vi "Grow bounding rectangle N pixels.vi"(4 "Bounding Rect":T1={"Left"=20.0, "Top"=30.0, "Right"=200.0, "Bottom"=300.0}, 5 "# pixels":dbl=10.0) -> (1 "Bounding Rect expanded":T1={"Left"=10.0, "Top"=20.0, "Right"=210.0, "Bottom"=310.0})   [LabVIEW 2013]
doc: "Grows outwardeach side of bounding rectangle by N pixels."
uses:
  Project Vis/Image Analysis/Analysis type defs/Bounding rectangle cluster.ctl
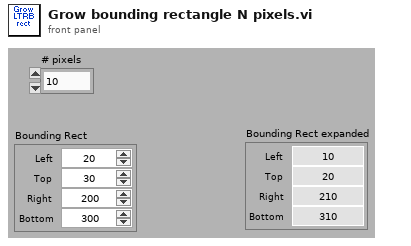
[diagram p1: front panel]
types:
  T1 = typedef "Bounding rectangle cluster.ctl" = cluster{"Left":dbl, "Top":dbl, "Right":dbl, "Bottom":dbl}
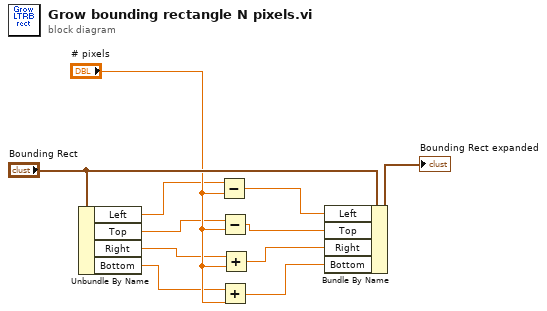
[diagram p0: block diagram]
diagram:
  n1 = Unbundle By Name("Bounding Rect") -> ("Left"=w8:dbl, "Top"=w7:dbl, "Right"=w6:dbl, "Bottom"=w5:dbl)
  n2 = Subtract(x=w8, y="# pixels") -> (x-y=w4:dbl)
  n3 = Subtract(x=w7, y="# pixels") -> (x-y=w3:dbl)
  n4 = Add(x=w5, y="# pixels") -> (x+y=w1:dbl)
  n5 = Add(x=w6, y="# pixels") -> (x+y=w2:dbl)
  n6 = Bundle By Name(cluster="Bounding Rect", "Left"=w4, "Top"=w3, "Right"=w2, "Bottom"=w1) -> (→"Bounding Rect expanded":T1)
